vi "toStringArray.vi"(8 "error in (no error)":errorcluster, 11 "ScriptEvent in":refnum<class "ScriptEvent.lvclass">) -> (0 "error out":errorcluster, 2 "eventStringArray":string[](array[string]), 3 "ScriptEvent out":refnum<class "ScriptEvent.lvclass">)   [LabVIEW 2009, in "Tools.lvlib" / "Scripting.lvlib" / "ScriptEvent.lvclass"]
uses:
  ScriptEvent.lvclass
  ScriptEvent.lvclass/ScriptEvent.ctl
  DatabaseHelpers/Database Objects/Channel/Channel.lvclass
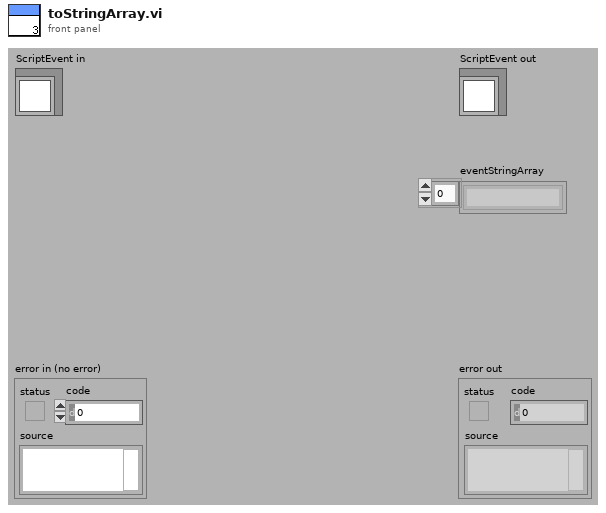
[diagram p1: front panel]
types:
  T1 = enum16{"Initialise", "MOT", "Molasses", "Optical Pumping", "Magnetic Trap", "RF Cooling", "Manipulation", "Switch Off", "Absorption Imaging", "Fluorscence Imaging", "Shut Down"}
  T2 = enum16{"changeValue", "pulse", "clock", "rampUp", "rampDown", "singleTone", "singleToneRamp", "playFile", "rf", "rfRamp"}
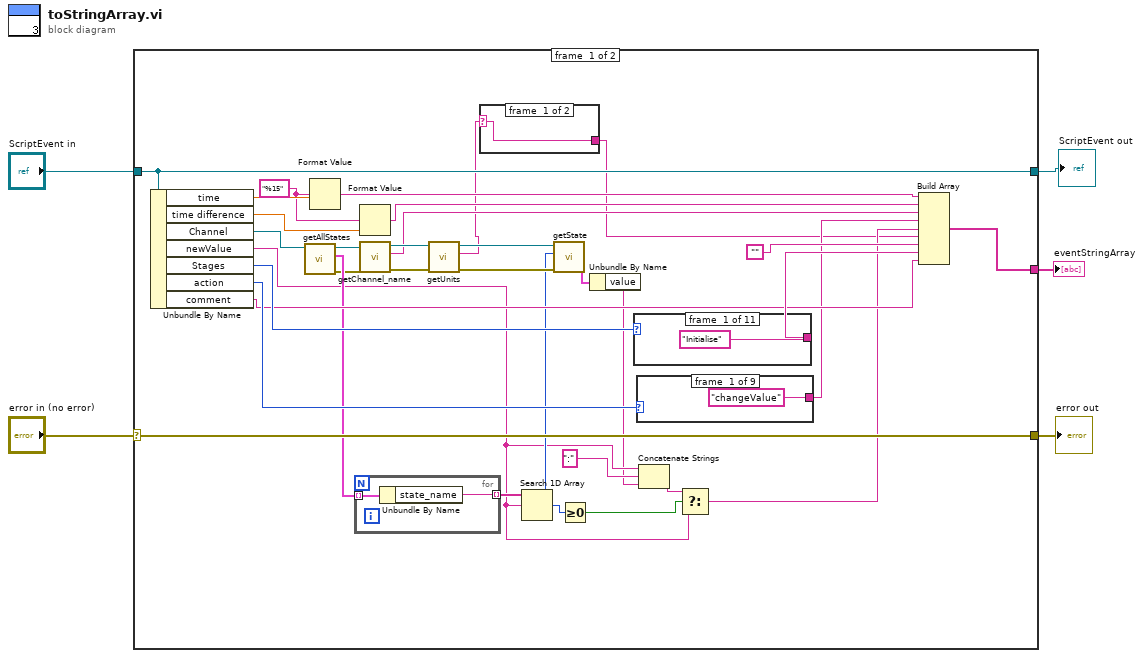
[diagram p0: block diagram]
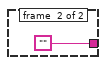
[diagram p2: hidden frame]
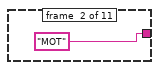
[diagram p3: hidden frame]
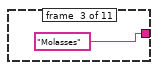
[diagram p4: hidden frame]
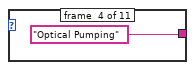
[diagram p5: hidden frame]
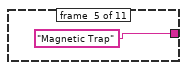
[diagram p6: hidden frame]
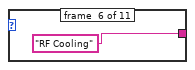
[diagram p7: hidden frame]
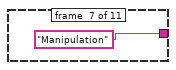
[diagram p8: hidden frame]
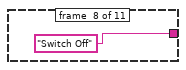
[diagram p9: hidden frame]
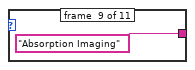
[diagram p10: hidden frame]
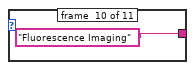
[diagram p11: hidden frame]
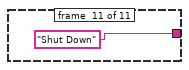
[diagram p12: hidden frame]
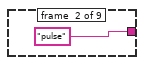
[diagram p13: hidden frame]
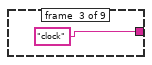
[diagram p14: hidden frame]
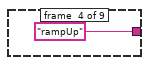
[diagram p15: hidden frame]
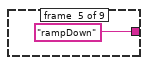
[diagram p16: hidden frame]
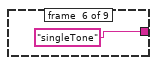
[diagram p17: hidden frame]
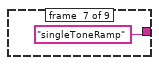
[diagram p18: hidden frame]
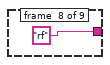
[diagram p19: hidden frame]
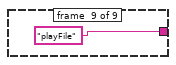
[diagram p20: hidden frame]
diagram:
  n1 = case shown="No Error" "error in (no error)" {
    selector: "error in (no error)" -> [w39 w65]
    tunnel: [w39 w65] -> w4
    tunnel: [w38 w64] -> w2
    tunnel: "ScriptEvent in" -> [w38 w64]
    tunnel: [w25 _] -> w1
    frame #0 {
      w35 = "%15"
      n2 = Unbundle By Name(w38) -> ("time"=w37:dbl, "time difference"=w36:dbl, "Channel"=w20:refnum<class "Channel.lvclass">, "newValue"=w9:string, "Stages"=w28:T1, "action"=w29:T2, "comment"=w26:string)
      n3 = call "getAllStates.vi"("Channel.lvclass in"=w20) -> ("error out"=w19:errorcluster, "states"=w22:cluster{"state_name":string, "value":string}[], "Channel.lvclass out"=w21:refnum<class "Channel.lvclass">)  [unwired: 8 in]
      n4 = Format Value(format string=w35, value (0)=w37) -> (output string=w32:string)  [unwired: 1 in]
      n5 = for {
        tunnel: w22 -> [w43] mode=indexing
        tunnel: [w42] -> w18 mode=indexing
        n6 = Unbundle By Name(w43) -> ("state_name"=w42:string)
      }
      n7 = Format Value(format string=w35, value (0)=w36) -> (output string=w31:string)  [unwired: 1 in]
      n8 = call "getChannel_name.vi"("error in (no error)"=w19, "Channel.lvclass in"=w21) -> ("error out"=w33:errorcluster, "channel_name"=w30:string, "Channel.lvclass out"=w34:refnum<class "Channel.lvclass">)  [unwired: 7 in]
      n9 = call-dynamic "getUnits.vi"("error in (no error)"=w33, "Channel.lvclass in"=w34) -> ("error out"=w12:errorcluster, "units"=w7:string, "Channel.lvclass out"=w13:refnum<class "Channel.lvclass">)  [unwired: 7 in]
      n10 = case shown="\"N-A\"" w7 {
        selector: w7 -> [w40 _]
        tunnel: [w40 ""] -> w6
        frame #0 {
        }
        frame #1 {
        }
      }
      n11 = Search 1D Array(1D array=w18, element=w9) -> (index of element=w11:i32)  [unwired: 1 in]
      n12 = call "getState.vi"("error in (no error)"=w12, "index"=w11, "Channel.lvclass in"=w13) -> ("state"=w10:cluster{"state_name":string, "value":string})  [unwired: 6 in, 2 out]
      n13 = Greater Or Equal To 0?(x=w11) -> (x >= 0?=w15:bool)
      n14 = Unbundle By Name(w10) -> ("value"=w8:string)
      n15 = case shown="\"Molasses\"" w28 {
        tunnel: ["Initialise" "MOT" "Molasses" "Optical Pumping" "Magnetic Trap" "RF Cooling" "Manipulation" "Switch Off" "Absorption Imaging" "Fluorescence Imaging" "Shut Down"] -> w27
        frame #0 {
        }
        frame #1 {
        }
        frame #2 {
        }
        frame #3 {
        }
        frame #4 {
        }
        frame #5 {
        }
        frame #6 {
        }
        frame #7 {
        }
        frame #8 {
        }
        frame #9 {
        }
        frame #10 {
        }
      }
      n16 = case shown="\"rf\"" w29 {
        tunnel: ["changeValue" "pulse" "clock" "rampUp" "rampDown" "singleTone" "singleToneRamp" "rf" "playFile"] -> w23
        frame #0 {
        }
        frame #1 {
        }
        frame #2 {
        }
        frame #3 {
        }
        frame #4 {
        }
        frame #5 {
        }
        frame #6 {
        }
        frame #7 {
        }
        frame #8 {
        }
      }
      n17 = Concatenate Strings(w9, ":", w8) -> (w16:string)
      n18 = Select(t=w16, s=w15, f=w9) -> (s? t:f=w14:string)
      n19 = Build Array(w32, w31, w30, w23, w14, w6, "", w27, w26) -> (w25:string[])
    }
    frame #1 {
    }
  }
  "error out" <- w4
  "ScriptEvent out" <- w2
  "eventStringArray" <- w1
